vi "dataProcess_peaks.vi"(0 "reference":refnum<class "OSA.lvclass">, 1 "X search full range":bool=TRUE, 7 "error in (no error)":errorcluster, 8 "X search min (/cm)":sgl format="%.2f", 9 "minPeakHeight (dB)":sgl format="%.2f", 12 "X search max (/cm)":sgl format="%.2f", 13 "thld (mW)":sgl format="%.2f", 15 "sorting (none)":enum16{"none", "position", "height", "width"}(ring)) -> (16 "peaks thld left":sgl[](array[numeric]), 18 "peaks thld right":sgl[](array[numeric]), 20 "duplicate reference":refnum<class "OSA.lvclass">, 21 "nr peaksFound":i32, 23 "peakCenter, (/cm)":sgl[](array[numeric]) format="%.2f", 24 "peakWidth, (/cm)":sgl[](array[numeric]) format="%.2f", 25 "peakHeight, (mW power absolute)":sgl[](array[numeric]) format="%.2f", 27 "error out":errorcluster)   [LabVIEW 2010, in "OSA.lvclass"]
doc: "Retrieves all peaks in the given data set between the given indices. The properties of the found peaks are stored in the given arrays peakCenter, peakWidth and peakHeight."
uses:
  OSA.lvclass
  typeDef/spectrum_y_unit.ctl
  FTSLib.dll
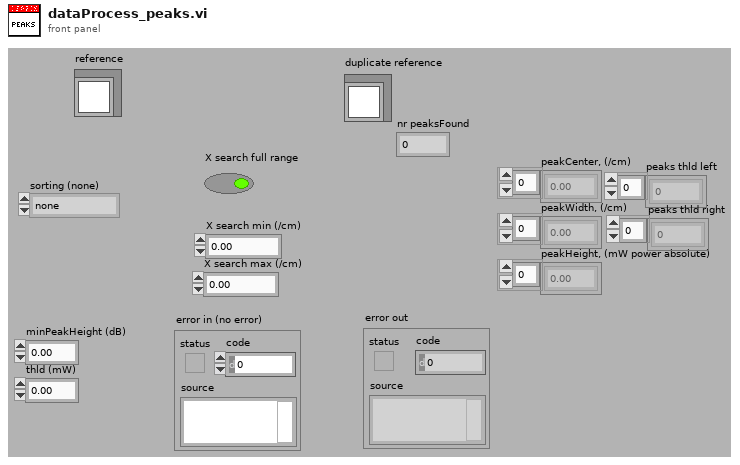
[diagram p1: front panel]
types:
  T1 = typedef "OSA.lvclass/spectrum_y_unit.ctl" = enum16{"dBm pwr absolute", "dBm pwr density", "mW pwr absolute", "mW pwr density"}
  T2 = enum16{"get", "init", "set interferogram", "set spectrum", "cleanUp"}
  T3 = typedef "OSA.lvclass/ObjectAttributes.ctl" = cluster{"Stop":bool, "dataType":T4, "spectrometerIdx":u16, "buffer size interferogram":i32, "interferogram":cluster{"new":bool, "plot_x_ min":sgl, "plot_x_max":sgl, "plot_y_min":sgl, "plot_y_max":sgl, "Graph Intrfrgrm":T5, "timeStamp":u32, "signal (%)":dbl, "traces":cluster{"idx":u32, "broadBand":bool, "monoChromatic":bool, "peakToPeakSignal":dbl, "peakToPeakPos":dbl}[], "traces idx last":i32, "contrast (%)":dbl}, "spectrum":cluster{"new":bool, "plot_x_min":sgl, "plot_x_max":sgl, "plot_unit_x":T6, "plot_unit_y":T7, "plot_y_min":sgl, "plot_y_max":sgl, "Graph Spectrum":T5, "timeStamp":u32, "X_VAL_OPTIONS":enum16{"MIN_MAX", "ARRAY"}, "traces":cluster{"idx":u32}[], "traces idx last":i32}, "Thorlabs_OSA_64.lvclass:queue_action.ctlqueue ref":refnum<queue>, "action":T8, "plot zoom step":dbl, "buffer semaphore":T9, "acq stopped":bool, "dataType active":T4, "temperature (degr C)":sgl, "pressure (hPa)":sgl, "rel humidity (%)":sgl, "settings":cluster{"resolution":u16, "sensitivity":u16, "Average":bool, "average nr":u32, "apodisation":T10, "acq delay (ms)":u32, "airMesure":T11, "wmtr on":bool, "intfgrm_smooth_width":u16, "intfgrm_smooth_nrOfPasses":u16, "intfgrm_smooth":T12, "phaseCorrection":T13, "zeroFill":u8, "spectr_smooth":T12, "spectr_smooth_width":u16, "spectr_smooth_nrOfPasses":u16, "resolution (/cm)":sgl, "REF wavelength, (nm)":dbl, "gain_idx":u16, "gainAuto":bool, "gain_relative":dbl, "PD sensitivity mode":T14, "PD senseMode implemented":bool, "SensorTemperature implemented":bool, "SensorPressure implemented":bool, "SensorHumidity implemented":bool, "attenuationAuto":bool, "attenuationOnOff":bool, "attenuationAvailable":bool, "offsetAvailable":bool, "offset":i32, "offset max":u16, "contrastAvailable":bool}, "peaks position":sgl[], "peaks width":sgl[], "peaks height":sgl[], "peaks max nr":u32, "peaks latest nr":i32, "peaks new":bool, "power":dbl, "power new":bool, "path":string, "wavelength (WNr)":dbl, "wavelength new":bool, "buffer size spectrum":i32, "status":string, "vi reference":refnum<vi>, "funcPointer":u64, "libraryPointer":u64, "singleAcquisition":bool, "coherenceLength (cm)":dbl, "coherenceLength new":bool, "spectrometer model":string, "spectrometer serial nr":string, "peaks thld left":sgl[], "peaks thld right":sgl[], "coherenceLength error (cm)":dbl, "ADC bits":u16, "peaks position centroid":sgl[], "peaks height centroid":sgl[], "OSA series":T15, "channel index spectrum":u16, "spectrometer rangeLow, (/cm)":dbl, "spectrometer rangeHigh, (/cm)":dbl, "channel index interferogram":u16, "virtualSource":bool}
  T4 = typedef "OSA.lvclass/acq_dataType.ctl" = enum16{"none", "interferogram", "spectrum"}
  T5 = typedef "OSA.lvclass/graph_intensity.ctl" = refnum<vi>
  T6 = typedef "OSA.lvclass/spectrum_x_unit.ctl" = enum16{"wavenr/cm", "THz", "eV", "nm_air", "nm_vac"}
  T7 = typedef "OSA.lvclass/y_unit.ctl" = enum16{"ADC counts", "dBm pwr absolute", "dBm pwr density", "mW pwr absolute", "mW pwr density"}
  T8 = typedef "OSA.lvclass/queue_action.ctl" = enum16{"none", "stop", "GUI_plotInterferogram", "GUI_plotSpectrum", "GUI_plotInterferogramRescale", "GUI_plotSpectrumRescale", "GUI_plotInterferogramReset", "GUI_plotSpectrumReset", "GUI_plotInterferogramAutoScaleY", "GUI_plotSpectrumAutoScaleY", "GUI_plotInterferogramZoomOut", "GUI_plotSpectrumZoomOut", "GUI_plotInterferogramPane", "GUI_plotSpectrumPane", "GUI_plotInterferogramZoomMouse", "GUI_plotSpectrumZoomMouse", "GUI_spectrumChannelType", "GUI_channel", "ENVIRONMENT temperature", "ENVIRONMENT pressure", "MODE_resolution set", "MODE_resolution get", "MODE_sensitivity set", "MODE_sensitivity get", "MODE_PDTemperature set", "MODE_PDTemperature get", "REBOOT/RESET firmware", "ACQASYNC_acquireSingleSpectrum", "ACQASYNC_continuous start", "ACQASYNC_continuous stop\n", "ACQASYNC_get last interferogram", "ACQASYNC_get last spectrum", "ACQASYNC_get last waveNr", "ACQOPT_interferogram smoothing set", "ACQOPT_interferogram smoothing get", "ACQOPT_spectrum smoothing set", "ACQOPT_spectrum smoothing get", "ACQOPT_apodisation type set", "ACQOPT_apodisation type get", "ACQOPT_phase correction type set", "ACQOPT_phase correction type get", "ACQOPT_acqIntervall_set", "ACQOPT_acqIntervall_get", "ACQOPT_average spectrum set", "ACQOPT_average spectrum get", "ACQOPT_rolling average set", "ACQOPT_rolling average get", "ACQOPT_zero fill factor set", "ACQOPT_zero fill factor get", "ACQOPT_cycle counting set", "ACQOPT_cycle counting get", "ACQOPT_air measure option set", "ACQOPT_air measure option get", "ACQOPT_gainLevel auto get", "ACQOPT_gainLevel auto set", "ACQOPT_gainLevel get", "ACQOPT_gainLevel set", "ACQOPT_offset set", "ACQOPT_attenuator_auto_set", "ACQOPT_attenuator_set", "ACQOPT_getAll", "INSTRUMENT_PROPERTY_range_WaveNr_min", "INSTRUMENT_PROPERTY_range_WaveNr_max", "INSTRUMENT_PROPERTY_reference_wavelength_cm^-1", "INSTRUMENT_PROPERTY_samplesPerRefPeriod", "INSTRUMENT_PROPERTY_resolution_waveNrPercm", "INSTRUMENT_PROPERTY_availableGainLevels", "INSTRUMENT_PROPERTY_status", "CONVERT", "ANALYSE_POWER", "ANALYSE_PEAKS", "ANALYSE_WAVELENGTH", "ANALYSE_SPECTRUM", "ANALYSE_INTERFEROGRAM", "ANALYSE_COHERENCE_LENGTH", "MATH", "MATH_power", "MATH_peaks", "FILE", "miscellaneous"}
  T9 = typedef "Semaphore RefNum" = refnum<k1>
  T10 = typedef "OSA.lvclass/apodisation.ctl" = enum16{"NONE", "NORTON_BEER_WEAK", "NORTON_BEER_MEDIUM", "NORTON_BEER_STRONG", "TRIANGULAR", "COSINE", "HANN", "HAMMING", "BLACKMANHARRIS3", "BLACKMANHARRIS4", "GAUSSIAN"}
  T11 = typedef "OSA.lvclass/airMeasure.ctl" = enum16{"TEMPERATURE", "PRESSURE"}
  T12 = typedef "OSA20X_misc.lvlib/interferogram_smoothing.ctl" = enum16{"NONE", "BINOMIAL", "SAVITSKY_GOLAY", "FOURIER", "MOVING_AVERAGE", "GAUSSIAN"}
  T13 = typedef "OSA.lvclass/phaseCorrection.ctl" = enum16{"NONE", "MERTZ", "FORMAN", "MERTZ_FILE", "FORMAN_FILE", "FUTURE COMP."}
  T14 = typedef "OSA20X_misc.lvlib/PDTemperatureMode.ctl" = enum16{"cool: better sensitivity/noise floor", "warm: extended wl range"}
  T15 = typedef "OSA.lvclass/OSA_series.ctl" = enum16{"OSA200", "OSA300", "UNKNOWN"}
  T16 = typedef "OSA.lvclass/spectrum_properties.ctl" = cluster{"length":u32, "X min":sgl, "X max":sgl, "X_VAL_OPTIONS":T17}
  T17 = typedef "OSA.lvclass/xVal_option.ctl" = enum16{"MIN_MAX", "ARRAY"}
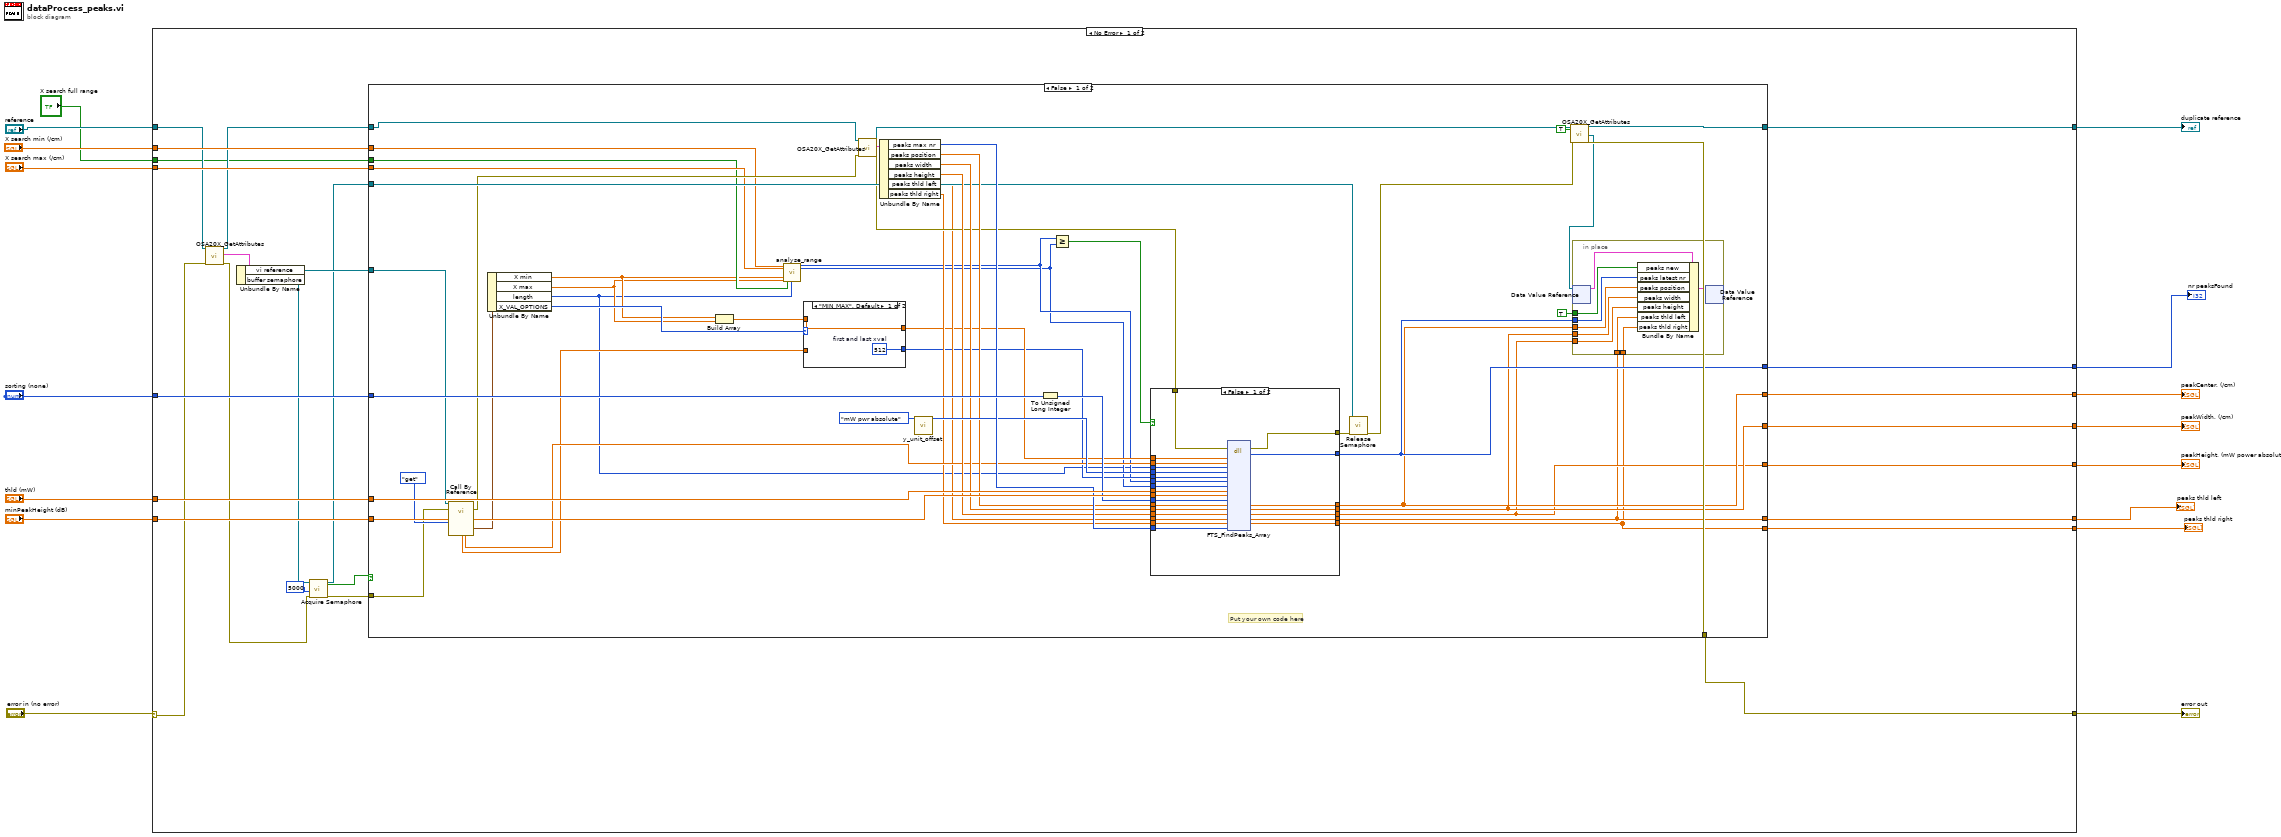
[diagram p0: block diagram]
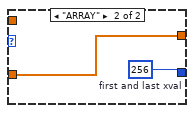
[diagram p2: hidden frame]
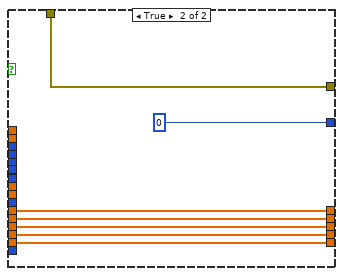
[diagram p3: hidden frame]
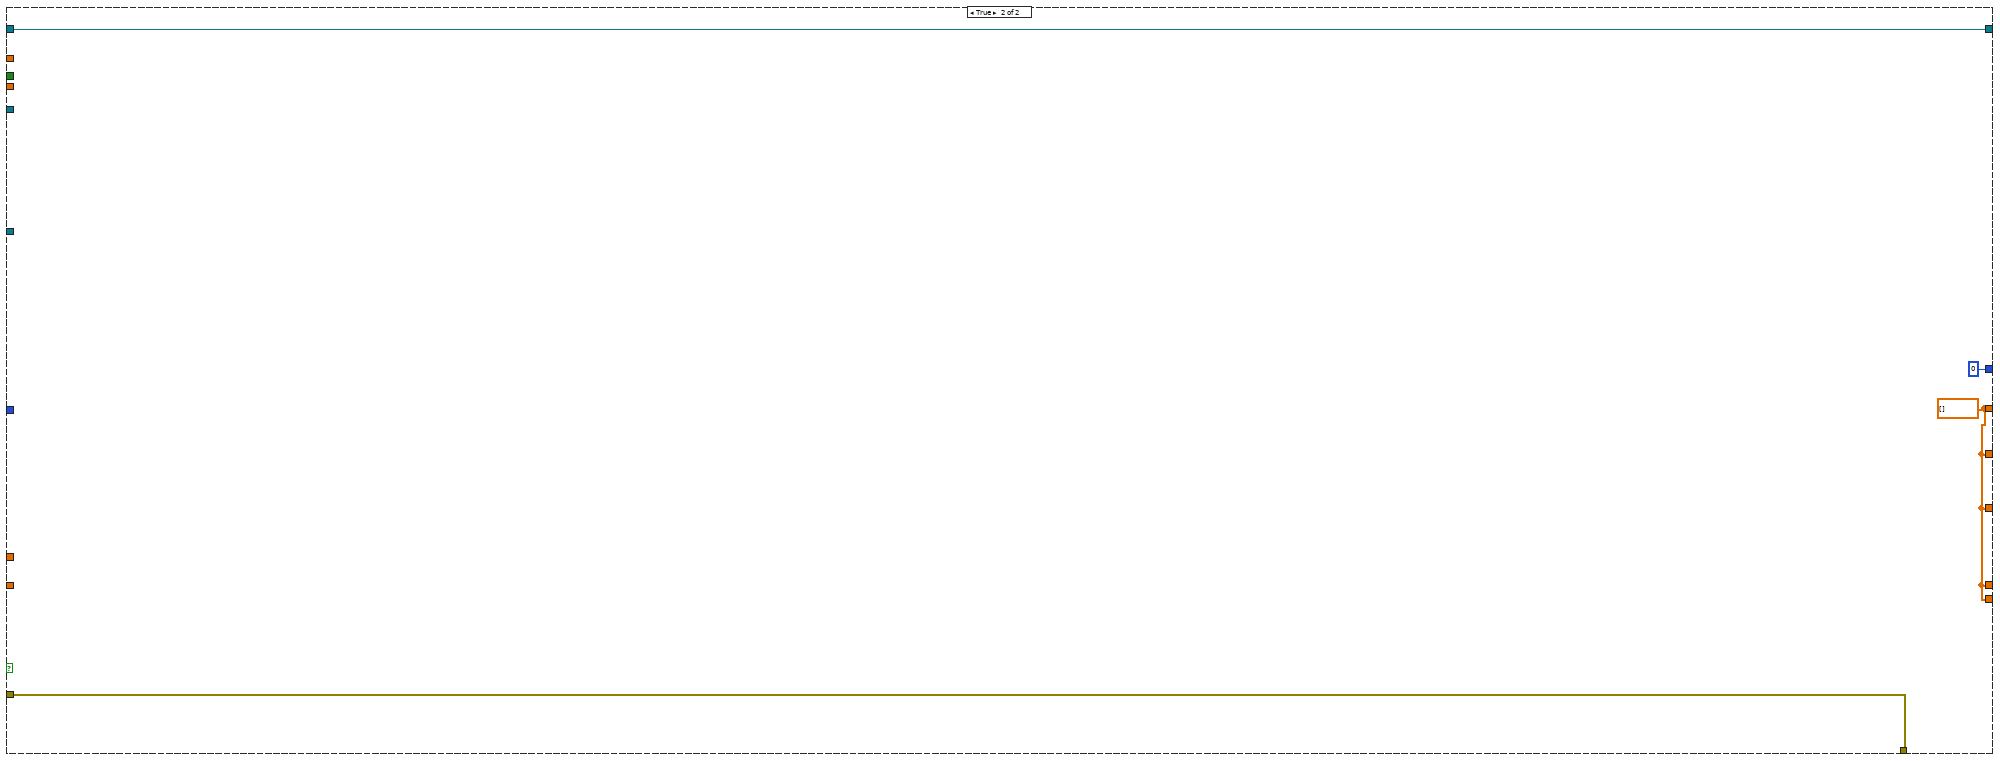
[diagram p4: hidden frame]
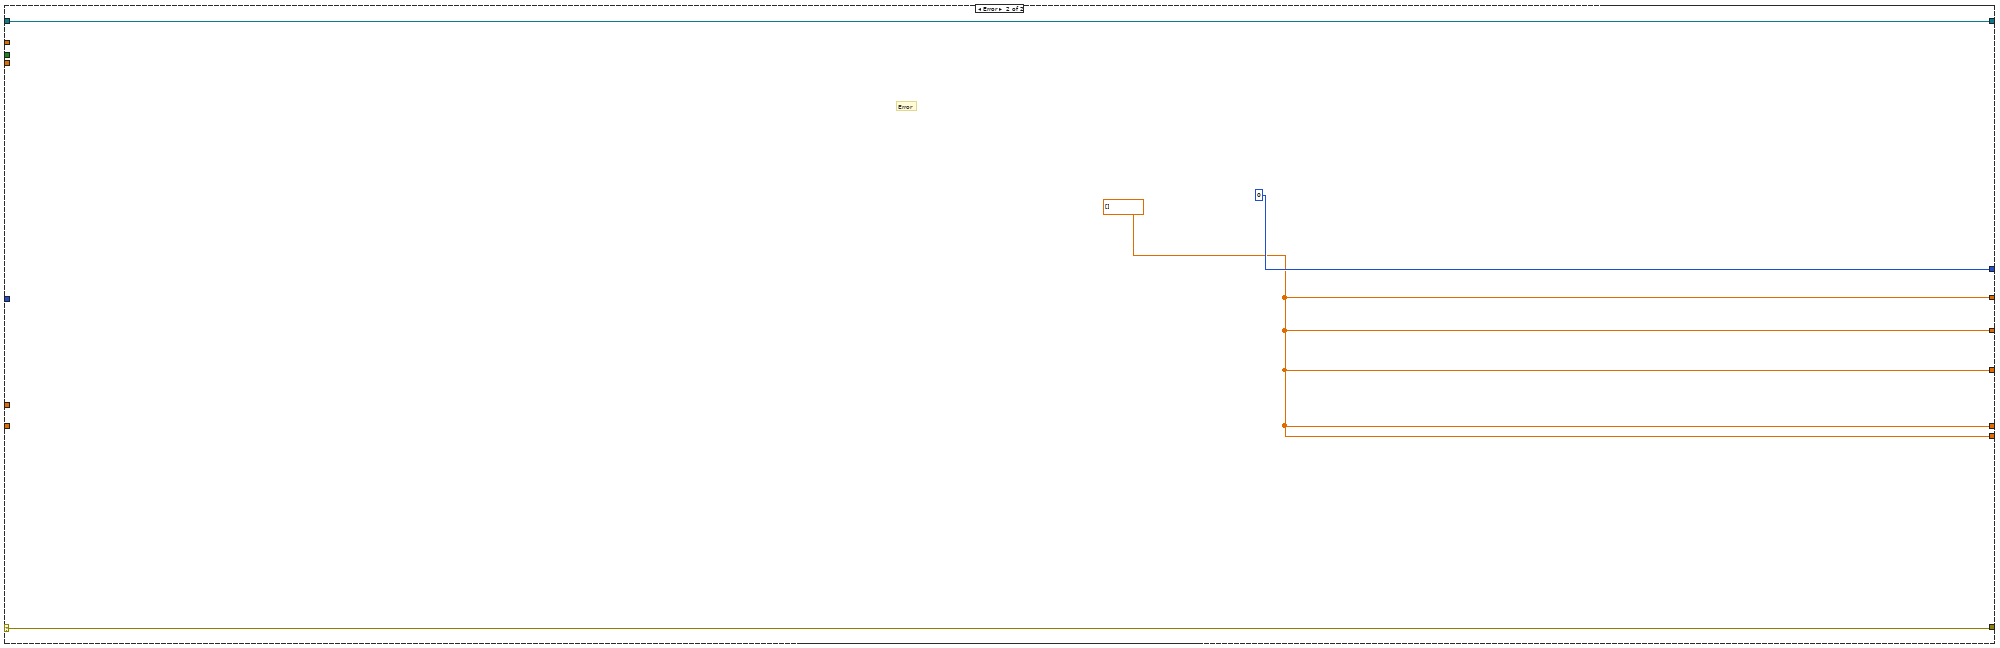
[diagram p5: hidden frame]
diagram:
  n1 = case shown="No Error" "error in (no error)" {
    selector: "error in (no error)" -> [w29 w142]
    tunnel: [w37 w142] -> w16
    tunnel: "reference" -> [w23 w143]
    tunnel: [w38 w143] -> w13
    tunnel: "minPeakHeight (dB)" -> [w41 _]
    tunnel: "thld (mW)" -> [w40 _]
    tunnel: "sorting (none)" -> [w39 _]
    tunnel: [w34 w140] -> w9
    tunnel: [w33 w140] -> w8
    tunnel: [w35 w140] -> w7
    tunnel: [w36 0] -> w6
    tunnel: "X search min (/cm)" -> [w32 _]
    tunnel: "X search max (/cm)" -> [w31 _]
    tunnel: [w19 w140] -> w3
    tunnel: [w18 w140] -> w2
    tunnel: "X search full range" -> [w17 _]
    frame No Error {
      n2 = call "OSA20X_GetAttributes.vi"("reference in"=w23, "error in (no error)"=w29) -> ("reference out"=w22:refnum<class "OSA.lvclass">, "Data"=w20:T3, "error out"=w28:errorcluster)  [unwired: 14 in, 1 out]
      n3 = Unbundle By Name(w20) -> ("vi reference"=w24:refnum<vi>, "buffer semaphore"=w26:T9)
      n4 = call <vilib>:"Acquire Semaphore.vi"("error in (no error)"=w28, "ms timeout (-1)"=5000, "semaphore"=w26) -> ("error out"=w27:errorcluster, "timed out"=w25:bool, "semaphore out"=w21:T9)  [unwired: 2 in]
      n5 = case shown="False" w25 {
        tunnel: w41 -> [w91 _]
        tunnel: w40 -> [w90 _]
        tunnel: w39 -> [w89 _]
        tunnel: w22 -> [w88 w138]
        tunnel: [w84 w138] -> w38
        tunnel: [w83 w137] -> w37
        tunnel: [w64 0 ("return type")] -> w36
        tunnel: [w61 w136] -> w35
        tunnel: [w63 w136] -> w34
        tunnel: [w62 w136] -> w33
        tunnel: w32 -> [w48 _]
        tunnel: w31 -> [w47 _]
        tunnel: w27 -> [w76 w137]
        tunnel: w24 -> [w75 _]
        tunnel: w21 -> [w70 _]
        tunnel: [w57 w136] -> w19
        tunnel: [w56 w136] -> w18
        tunnel: w17 -> [w46 _]
        frame False {
          # "Put your own code here"
          n6 = call-by-ref "?"(reference=w75, error in=w76, "action"=T2."get") -> (error out=w69:errorcluster, "spectrum X"=w54:sgl[], "spectrum Y"=w74:sgl[], "spectrum prop"=w73:T16)  [unwired: 14 in, 3 out]
          n7 = Unbundle By Name(w73) -> ("X min"=w44:sgl, "X max"=w43:sgl, "length"=w42:u32, "X_VAL_OPTIONS"=w51:T17)
          n8 = Build Array(w44, w43) -> (w45:sgl[])
          n9 = call "analyse_range.vi"("X search min (/cm)"=w48, "X search max (/cm)"=w47, "X min"=w44, "X max"=w43, "full range"=w46, "length"=w42) -> ("index start"=w50:u32, "index stop"=w49:u32)  [unwired: 12 in]
          n10 = case shown="\"MIN_MAX\", Default" w51 {
            tunnel: w54 -> [_ w95]
            tunnel: [w93 w95] -> w53
            tunnel: w45 -> [w93 _]
            tunnel: [w92 w94] -> w52
            frame "MIN_MAX", Default {
              w92 = u32 512  # first and last xval
            }
            frame "ARRAY" {
              w94 = u32 256  # first and last xval
            }
          }
          n11 = call "OSA20X_GetAttributes.vi"("reference in"=w88, "error in (no error)"=w69) -> ("reference out"=w85:refnum<class "OSA.lvclass">, "Data"=w67:T3, "error out"=w60:errorcluster)  [unwired: 14 in, 1 out]
          n12 = Unbundle By Name(w67) -> ("peaks max nr"=w86:u32, "peaks position"=w80:sgl[], "peaks width"=w79:sgl[], "peaks height"=w78:sgl[], "peaks thld left"=w59:sgl[], "peaks thld right"=w58:sgl[])
          n13 = call "y_unit_offset.vi"("spectrum y unit (mW pwr absolute)"=spectrum_y_unit."mW pwr absolute") -> ("yUnit val"=w82:i32)  [unwired: 18 in]
          n14 = To Unsigned Long Integer(number=w89) -> (unsigned 32bit integer=w87:u32)
          n15 = Greater Or Equal?(x=w50, y=w49) -> (x >= y?=w81:bool)
          n16 = case shown="False" w81 {
            tunnel: w91 -> [w128 _]
            tunnel: w90 -> [w127 _]
            tunnel: w87 -> [w126 _]
            tunnel: w80 -> [w125 w134]
            tunnel: w79 -> [w124 w133]
            tunnel: w78 -> [w123 w132]
            tunnel: w86 -> [w122 _]
            tunnel: [w121 0] -> w64
            tunnel: w74 -> [w120 _]
            tunnel: [w119 w132] -> w61
            tunnel: [w118 w134] -> w63
            tunnel: [w117 w133] -> w62
            tunnel: w82 -> [w116 _]
            tunnel: w52 -> [w115 _]
            tunnel: w53 -> [w114 _]
            tunnel: w42 -> [w113 _]
            tunnel: w50 -> [w112 _]
            tunnel: w49 -> [w111 _]
            tunnel: [w109 w131] -> w72
            tunnel: w60 -> [w110 w131]
            tunnel: w59 -> [w108 w130]
            tunnel: w58 -> [w107 w129]
            tunnel: [w106 w130] -> w57
            tunnel: [w105 w129] -> w56
            frame False {
              n17 = dll-call lib="FTSLib.dll" fn="FTS_FindPeaks_Array"(error in=w110, "xData"=w114, "yData"=w120, "length"=w113, "yAxisUnit"=w116, "xValueOption"=w115, "idxStart"=w112, "idxStop"=w111, "thld"=w127, "minPeakHeight_dB"=w128, "option"=w126, "peakCenter"=w125, "peakWidth"=w124, "peakHeight"=w123, "peakLeftPt"=w108, "peakRightPt"=w107, "maxPeaks"=w122) -> (error out=w109:errorcluster, "return type"=w121:i32, "peakCenter"=w118:sgl[], "peakWidth"=w117:sgl[], "peakHeight"=w119:sgl[], "peakLeftPt"=w106:sgl[], "peakRightPt"=w105:sgl[])  [unwired: 13 in, 1 out]
            }
            frame True {
            }
          }
          n18 = call <vilib>:"Release Semaphore.vi"("error in (no error)"=w72, "semaphore"=w70) -> ("error out"=w71:errorcluster)  [unwired: 4 in, 1 out]
          n19 = call "OSA20X_GetAttributes.vi"("reference in"=w85, "OnlyGetDvrReference(False)"=TRUE, "error in (no error)"=w71) -> ("reference out"=w84:refnum<class "OSA.lvclass">, "DataRef"=w66:refnum<data-value>, "error out"=w83:errorcluster)  [unwired: 13 in, 1 out]
          n20 = in-place {
            in-place-border: TRUE ("peaks new") -> [w103]
            in-place-border: w64 -> [w102]
            in-place-border: w63 -> [w101]
            in-place-border: w62 -> [w100]
            in-place-border: w61 -> [w99]
            in-place-border: w57 -> [w97]
            in-place-border: w56 -> [w96]
            n21 = in-place-dvr #1(w66) -> (w104:T3)  [unwired: 1 out]
            n22 = Bundle By Name(cluster=w104, "peaks new"=w103, "peaks latest nr"=w102, "peaks position"=w101, "peaks width"=w100, "peaks height"=w99, "peaks thld left"=w97, "peaks thld right"=w96) -> (w98:T3)
            n23 = in-place-dvr #1(w98) -> ()  [unwired: 2 out]
          }
        }
        frame True {
          w136 = sgl[] [] ("peaks position")
        }
      }
    }
    frame Error {
      w140 = sgl[] [] ("peakCenter")
      # "Error"
    }
  }
  "error out" <- w16
  "duplicate reference" <- w13
  "peakCenter, (/cm)" <- w9
  "peakWidth, (/cm)" <- w8
  "peakHeight, (mW power absolute)" <- w7
  "nr peaksFound" <- w6
  "peaks thld left" <- w3
  "peaks thld right" <- w2
